vi "2P_AdapUprite_Linlin.vi"() -> ()   [LabVIEW 2015] (continued)
                            n110 = local read "AI channels"() -> (w2310:i32[])
                            n111 = local read "CI channels"() -> (w2309:i32[])
                            n112 = call "2pparameters.vi"("command"="get") -> ("params out"=w2307:T12)  [unwired: 1 in]
                            n113 = Bundle By Name(cluster=w2307, "aAI"=w2310, "aCI"=w2309, "aAS"=w2304) -> (w2308:T12)
                            n114 = call "2pparameters.vi"("Params in"=w2308, "command"="set") -> ()  [unwired: 1 out]
                          }
                          frame #1 {
                            n115 = local read "Vy-min ref"() -> (w2315:dbl)
                            n116 = local read "Vy-max ref"() -> (w2316:dbl)
                            n117 = local read "Angle ref"() -> (w2314:dbl)
                            n118 = local read "Vx-min ref"() -> (w2317:dbl)
                            n119 = local write "counts"(0 ("counts")) -> ()
                            n120 = local write "graphtab"(T8."image" ("graphtab")) -> ()
                            n121 = local read "Vx-max ref"() -> (w2318:dbl)
                            n122 = property on="Stop" class="Bool (strict)"("Visible"=TRUE, "DisabledEnum"=T7."Enabled" ("Disabled")) -> ()  [unwired: 2 in, 2 out]
                            n123 = property on="Start" class="Bool (strict)"("Visible"=FALSE, "DisabledEnum"=T7."Disabled and Grayed Out" ("Disabled")) -> ()  [unwired: 2 in, 2 out]
                            n124 = script code="Xic=(ximax+ximin)./2;\nYic=(yimax+yimin)./2;\nximin=ximin-Xic;\nymin=ymin-Yic;\nxirmin=ximin.*cos(pi/180.*phi)+yimin.*sin(pi./180.*phi)+Xic;\nyirmin=-ximin.*sin(pi./180.*phi)+yimin.*cos(pi./180.*phi)+Yic;"("ximax"=w2318, "ximin"=w2317, "yimax"=w2316, "yimin"=w2315, "phi"=w2314) -> ("xirmin"=w2313:dbl, "yirmin"=w2312:dbl)  [unwired: 1 in, 1 out]
                            n125 = stacked-sequence {
                              tunnel: w2311 -> [_ w2343 _]
                              frame #0 {
                                n126 = local read "Measurement"() -> (w2325:T4)
                                n127 = case shown="\"X-Y-Z stack\"" w2325 {
                                frame "X-Y-t movie", Default {
                                n128 = call "2pparameters.vi"("command"="get") -> ("params out"=w2328:T12)  [unwired: 1 in]
                                n129 = Bundle By Name(cluster=w2328, "type"="X-Y-t movie") -> (w2326:T12)
                                n130 = call "2pparameters.vi"("Params in"=w2326, "command"="set") -> ()  [unwired: 1 out]
                                }
                                frame "X-Y-Z stack" {
                                n131 = call "2pparameters.vi"("command"="get") -> ("params out"=w2333:T12)  [unwired: 1 in]
                                n132 = Bundle By Name(cluster=w2333, "type"="X-Y-Z stack") -> (w2331:T12)
                                n133 = call "2pparameters.vi"("Params in"=w2331, "command"="set") -> ()  [unwired: 1 out]
                                }
                                frame "Lifetime (scan)" {
                                n134 = call "2pparameters.vi"("command"="get") -> ("params out"=w2338:T12)  [unwired: 1 in]
                                n135 = Bundle By Name(cluster=w2338, "type"="Lifetime (scan)") -> (w2336:T12)
                                n136 = call "2pparameters.vi"("Params in"=w2336, "command"="set") -> ()  [unwired: 1 out]
                                }
                                }
                              }
                              frame #1 {
                                n137 = Format Date/Time String(time format string (%c)="%Y%m%d", seconds (now)=w2343) -> (date/time string=w2342:string)  [unwired: 1 in]
                                n138 = Format Date/Time String(time format string (%c)="%H%M%S", seconds (now)=w2343) -> (date/time string=w2341:string)  [unwired: 1 in]
                                n139 = call "2pparameters.vi"("command"="get") -> ("params out"=w2347:T12)  [unwired: 1 in]
                                n140 = Bundle By Name(cluster=w2347, "date"=w2342, "time"=w2341) -> (w2346:T12)
                                n141 = call "2pparameters.vi"("Params in"=w2346, "command"="set") -> ()  [unwired: 1 out]
                              }
                              frame #2 {
                                n142 = call "configuration_2P_Linlin.vi"("command"="get") -> ("config out"=w2350:T14)  [unwired: 2 in, 1 out]
                                n143 = Unbundle By Name(w2350) -> ("CI names"=w2358:string[], "AI names"=w2359:string[])
                                n144 = call "2pparameters.vi"("command"="get") -> ("params out"=w2355:T12)  [unwired: 1 in]
                                n145 = Unbundle By Name(w2355) -> ("aCI"=w2356:i32[], "aAI"=w2357:i32[])
                                n146 = for {
                                tunnel: w2356 -> [w2369] mode=indexing
                                tunnel: w2358 -> [w2370]
                                tunnel: [w2368] -> w2360 mode=indexing
                                n147 = Index Array(array=w2370, index=w2369) -> (element=w2368:string)
                                }
                                n148 = for {
                                tunnel: w2357 -> [w2366] mode=indexing
                                tunnel: w2359 -> [w2367]
                                tunnel: [w2365] -> w2361 mode=indexing
                                n149 = Index Array(array=w2367, index=w2366) -> (element=w2365:string)
                                }
                                n150 = Build Array (concatenate)(w2360, w2361) -> (w2353:string[])
                                n151 = for {
                                tunnel: w2353 -> [w2363] mode=indexing
                                tunnel: [w2362] -> w2352 mode=indexing
                                i -> [w2364]
                                n152 = Bundle("String"=w2363, w2364) -> (w2362:cluster{"String":string, i32})  [unwired: 1 in]
                                }
                                n153 = property on="image2list" class="Ring (strict)"("StringsAndValues[]"=w2352) -> ()  [unwired: 2 in, 2 out]
                                n154 = property on="image1list" class="Ring (strict)"("StringsAndValues[]"=w2352) -> ()  [unwired: 2 in, 2 out]
                                n155 = property on="image1list chB" class="Ring (strict)"("StringsAndValues[]"=w2352) -> ()  [unwired: 2 in, 2 out]
                                n156 = property on="image1list chA" class="Ring (strict)"("StringsAndValues[]"=w2352) -> ()  [unwired: 2 in, 2 out]
                              }
                            }
                            n157 = call "setposition.vi"("Vy"=w2312, "Vx"=w2313) -> ()  [unwired: 1 in]
                          }
                          frame #2 {
                            n158 = call "X-array-databuffer.vi"("command"=enum16{"get", "set", "clear", "append"}."clear") -> ()  [unwired: 3 in, 2 out]
                            n159 = call "Y-array-databuffer.vi"("command"=enum16{"get", "set", "clear", "append"}."clear") -> ()  [unwired: 3 in, 2 out]
                            n160 = call "2pparameters.vi"("command"="get") -> ("params out"=w2374:T12)  [unwired: 1 in]
                            n161 = Unbundle By Name(w2374) -> ("aAS"=w2371:u32[], "autoshutter"=w2375:bool, "auto OD"=w2372:bool)
                            n162 = call "allAI-temp_img.vi"("command"=enum16{"get", "set", "clear", "append"}."clear") -> ()  [unwired: 3 in, 2 out]
                            n163 = case shown="True" w2372 {
                              frame False {
                              }
                              frame True {
                                n164 = call "configuration_2P_Linlin.vi"("command"="get") -> ("config out"=w2381:T14)  [unwired: 2 in, 1 out]
                                n165 = Unbundle By Name(w2381) -> ("image OD"=w2384:u16)
                                n166 = local read "ODfilt"() -> (w2383:u16)
                                n167 = call "filterwheelcontrol_nothorlabslib.vi"("Current OD filt"=w2383, "New ODfilt"=w2384) -> ()  [unwired: 1 in]
                              }
                            }
                            n168 = case shown="True" w2375 {
                              tunnel: w2371 -> [_ w2385]
                              frame False {
                              }
                              frame True {
                                n169 = call "shuttercontrol_multi.vi"("Autoshutter Chans"=w2385, "command"="close") -> ()  [unwired: 1 in, 1 out]
                              }
                            }
                            n170 = call "CH1-temp.vi"("command"=enum16{"get", "set", "clear", "add row"}."clear") -> ()  [unwired: 3 in, 2 out]
                            n171 = call "CH2-temp.vi"("command"=enum16{"get", "set", "clear", "add row"}."clear") -> ()  [unwired: 3 in, 2 out]
                          }
                          frame #3 {
                            n172 = local read "avpp"() -> (w2419:i32)
                            n173 = local read "Angle ref"() -> (w2418:dbl)
                            n174 = local read "ROI Type"() -> (w2417:u16)
                            n175 = local read "xpixels ref"() -> (w2414:i32)
                            n176 = local read "Vx-min ref"() -> (w2413:dbl)
                            n177 = local read "Vx-max ref"() -> (w2412:dbl)
                            n178 = local read "ypixels ref"() -> (w2410:i32)
                            n179 = local read "Vy-min ref"() -> (w2411:dbl)
                            n180 = local read "Vy-max ref"() -> (w2407:dbl)
                            n181 = local read "Sampling rate"() -> (w2401:dbl)
                            n182 = local read "finite samples"() -> (w2402:bool)
                            n183 = local read "continuous"() -> (w2405:bool)
                            n184 = local read "wavdet"() -> (w2406:bool)
                            n185 = local read "# of frames"() -> (w2404:i32)
                            n186 = local read "maxbufferAI"() -> (w2403:i32)
                            n187 = local read "Override AI buffer"() -> (w2387:bool)
                            n188 = call "2pparameters.vi"("command"="get") -> ("params out"=w2416:T12)  [unwired: 1 in]
                            n189 = Bundle By Name(cluster=w2416, "avpp"=w2419, "Angle Img"=w2418, "Xpixels Img"=w2414, "Vx-min Img"=w2413, "VX-max Img"=w2412, "Ypixels Img"=w2410, "Vy-min Img"=w2411, "Vy-max Img"=w2407, "srate"=w2401, "srate Img"=w2401, "finite"=w2402, "cont"=w2405, "wavdet"=w2406, "measpoints"=w2404, "maxbufferAI"=w2403, "Drawing Mode"=w2417, "Vz-reset"=0.0, "AIoverride"=w2387) -> (w2408:T12)
                            n190 = call "2pparameters.vi"("Params in"=w2408, "command"="set") -> ()  [unwired: 1 out]
                            n191 = local read "Vholding (mV)"() -> (w2390:sgl)
                            n192 = local read "OCgain"() -> (w2391:sgl)
                            n193 = local read "holdon"() -> (w2389:bool)
                            n194 = local read "Current Clamp"() -> (w2396:bool)
                            n195 = local read "Voltage Clamp"() -> (w2395:bool)
                            n196 = local read "CC_ICgain"() -> (w2394:dbl)
                            n197 = call "patchparameters.vi"("command"="get") -> ("Params out"=w2398:T16)  [unwired: 1 in]
                            n198 = Bundle By Name(cluster=w2398, "VC"=w2395, "CC"=w2396, "CC_icg (pA/mv)"=w2394, "VC_icg (mV/mV)"=sgl 10.0, "OCG (mV/pA)"=w2391, "OVG (mV/mV)"=0.1, "Vhold (mV)"=w2390, "holdon"=w2389) -> (w2397:T16)
                            n199 = call "patchparameters.vi"("Params in"=w2397, "command"="set") -> ()  [unwired: 1 out]
                          }
                          frame #4 {
                            # "these store the actual scanning waveforms (for one iteration)"
                            # "Generate Waveforms for Scanning Mirrors"
                            # "Creates The scanning waveform here"
                            n200 = call "2pparameters.vi"("command"="get") -> ("params out"=w2434:T12)  [unwired: 1 in]
                            n201 = Unbundle By Name(w2434) -> ("srate Img"=w2433:sgl, "Angle Img"=w2432:dbl, "VX-max Img"=w2431:dbl, "Vx-min Img"=w2430:dbl, "Xpixels Img"=w2429:i32, "Ypixels Img"=w2428:i32, "Vy-max Img"=w2427:dbl, "Vy-min Img"=w2426:dbl, "Drawing Mode"=w2425:u16)
                            n202 = call "ROI-databuffer.vi"("command"=enum16{"get", "set", "clear", "append"}."get") -> ("array out"=w2424:cluster{"x":sgl, "y":sgl}[])  [unwired: 4 in]
                            n203 = call "ScanningWaveform_v4.vi"("Vy-min"=w2426, "Vy-max"=w2427, "yPixels/tPixels"=w2428, "xPixels/rPixels"=w2429, "Vx-min"=w2430, "Vx-max"=w2431, "Drawing Mode"=w2425, "Angle"=w2432, "AOrate"=w2433, "Points"=w2424) -> ("numPixels"=w2420:dbl, "Y-WaveArray"=w2423:dbl[], "P"=w2421:dbl, "X-WaveArray"=w2422:dbl[])  [unwired: 6 in]
                            n204 = call "2pparameters.vi"("command"="get") -> ("params out"=w2442:T12)  [unwired: 1 in]
                            n205 = call "Y-array-databuffer.vi"("array in"=w2423, "command"=enum16{"get", "set", "clear", "append"}."set") -> ()  [unwired: 2 in, 2 out]
                            n206 = call "X-array-databuffer.vi"("array in"=w2422, "command"=enum16{"get", "set", "clear", "append"}."set") -> ()  [unwired: 2 in, 2 out]
                            n207 = Bundle By Name(cluster=w2442, "P"=w2421, "sAOxy"=w2420) -> (w2439:T12)
                            n208 = call "2pparameters.vi"("Params in"=w2439, "command"="set") -> ()  [unwired: 1 out]
                          }
                          frame #5 {
                            # "rem2Ps"
                            # "A2Ps"
                            # "Al"
                            # "Rl"
                            # "Combines scanning waveform with \"wavform generation\" waveforms"
                            n209 = stacked-sequence {
                              seq-local: [w2461 _ _ _ _ _ _ _ _ _ _] -> [_ w2581 _ w2636 _ w2716 _ _ _ _ _]
                              seq-local: [w2462 _ _ _ _ _ _ _ _ _ _] -> [_ w2582 w2592 _ w2685 _ _ _ _ _ _]
                              seq-local: [_ _ w2591 _ _ _ _ _ _ _ _] -> [_ _ _ _ w2679 _ _ _ _ _ _]
                              seq-local: [_ _ _ w2635 _ _ _ _ _ _ _] -> [_ _ _ _ _ w2715 _ _ _ _ _]
                              seq-local: [w2458 _ _ _ _ _ _ _ _ _ _] -> [_ w2578 _ _ _ _ _ _ w2925 w2993 _]
                              seq-local: [w2457 _ _ _ _ _ _ _ _ _ _] -> [_ w2577 _ _ _ _ _ _ w2926 w2994 _]
                              seq-local: [w2464 _ _ _ _ _ _ _ _ _ _] -> [_ _ _ _ _ _ w2754 _ w2924 w2992 _]
                              seq-local: [w2460 _ _ _ _ _ _ _ _ _ _] -> [_ w2576 _ _ _ _ w2753 w2832 _ _ _]
                              seq-local: [w2459 _ _ _ _ _ _ _ _ _ _] -> [_ w2575 _ _ _ _ w2752 w2831 _ _ _]
                              seq-local: [w2463 _ _ _ _ _ _ _ _ _ _] -> [_ _ _ _ _ _ w2751 w2830 _ _ _]
                              tunnel: [_ _ w2590 _ _ _ _ _ _ _ _] -> w2455
                              tunnel: [_ _ w2589 _ _ _ _ _ _ _ _] -> w2454
                              tunnel: [w2462 _ _ _ _ _ _ _ _ _ _] -> w2456
                              tunnel: [w2461 _ _ _ _ _ _ _ _ _ _] -> w2453
                              tunnel: [_ _ _ w2634 _ _ _ _ _ _ _] -> w2452
                              tunnel: [_ _ _ w2633 _ _ _ _ _ _ _] -> w2451
                              tunnel: [w2460 _ _ _ _ _ _ _ _ _ _] -> w2450
                              tunnel: [w2459 _ _ _ _ _ _ _ _ _ _] -> w2449
                              tunnel: [_ _ _ _ _ _ w2750 _ _ _ _] -> w2448
                              tunnel: [_ _ _ _ _ _ _ w2829 _ _ _] -> w2447
                              tunnel: [w2458 _ _ _ _ _ _ _ _ _ _] -> w2446
                              tunnel: [w2457 _ _ _ _ _ _ _ _ _ _] -> w2445
                              tunnel: [_ _ _ _ _ _ _ _ w2923 _ _] -> w2444
                              tunnel: [_ _ _ _ _ _ _ _ _ w2991 _] -> w2443
                              frame #0 {
                                # "channels\nadded/removed"
                                # "all these arrows go to frames\n6 and 7"
                                # "for a next version, give ome thought to\nthe possibilit of intermittently updating the\nwaveforms. it will have to be a calculation\nbased on speed of CPU and program on the one hand\nand length of measurement on the other. but then it should be possible, in principle, to \nupdate the waveform on the fly and that way cut up a longer measurement in smaller parts."
                                # "Y"
                                # "X"
                                # "This frame takes channels from \"waveform generation\" and adds, X,Y,2p shutter and Lifetime Timestamp (if those where not manually defined in WG)"
                                n210 = stacked-sequence {
                                tunnel: [w2467 _ _ _] -> w2462
                                tunnel: [_ w2479 _ _] -> w2461
                                tunnel: [_ _ _ w2542] -> w2457
                                tunnel: [_ _ _ w2541] -> w2458
                                tunnel: [_ _ _ w2540] -> w2464
                                tunnel: [_ _ w2492 _] -> w2460
                                tunnel: [_ _ w2491 _] -> w2459
                                tunnel: [_ _ w2490 _] -> w2463
                                frame #0 {
                                n211 = call "configuration_2P_Linlin.vi"("command"="get") -> ("config out"=w2465:T14)  [unwired: 2 in, 1 out]
                                n212 = Unbundle By Name(w2465) -> ("Voltage to Xgalvo"=w2468:i32)
                                n213 = call "2pparameters.vi"("command"="get") -> ("params out"=w2471:T12)  [unwired: 1 in]
                                n214 = in-place {
                                in-place-border: w2468 -> [w2476]
                                in-place-border: [w2473] -> w2467
                                n215 = in-place-cluster #1(w2471) -> ("aAO"=w2475:u32[])
                                n216 = call "add channel to active arrayv2.vi"("line array in"=w2475, "line to add"=w2476) -> ("line array out"=w2474:u32[], "addition"=w2473:bool)  [unwired: 1 out]
                                n217 = in-place-cluster #1("aAO"=w2474) -> (w2469:T12)
                                }
                                n218 = call "2pparameters.vi"("Params in"=w2469, "command"="set") -> ()  [unwired: 1 out]
                                }
                                frame #1 {
                                n219 = call "configuration_2P_Linlin.vi"("command"="get") -> ("config out"=w2477:T14)  [unwired: 2 in, 1 out]
                                n220 = Unbundle By Name(w2477) -> ("Voltage to Ygalvo"=w2480:i32)
                                n221 = call "2pparameters.vi"("command"="get") -> ("params out"=w2483:T12)  [unwired: 1 in]
                                n222 = in-place {
                                in-place-border: w2480 -> [w2488]
                                in-place-border: [w2485] -> w2479
                                n223 = in-place-cluster #2(w2483) -> ("aAO"=w2487:u32[])
                                n224 = call "add channel to active arrayv2.vi"("line array in"=w2487, "line to add"=w2488) -> ("line array out"=w2486:u32[], "addition"=w2485:bool)  [unwired: 1 out]
                                n225 = in-place-cluster #2("aAO"=w2486) -> (w2481:T12)
                                }
                                n226 = call "2pparameters.vi"("Params in"=w2481, "command"="set") -> ()  [unwired: 1 out]
                                }
                                frame #2 {
                                n227 = call "2pparameters.vi"("command"="get") -> ("params out"=w2494:T12)  [unwired: 1 in]
                                n228 = Unbundle By Name(w2494) -> ("autoshutter"=w2493:bool, "wavdet"=w2489:bool)
                                n229 = case shown="False" w2493 {
                                tunnel: [w2499 w2522] -> w2492
                                tunnel: [w2498 FALSE ("removal")] -> w2491
                                tunnel: [w2497 w2521] -> w2490
                                tunnel: w2489 -> [w2496 _]
                                frame False {
                                n230 = case shown="False" w2496 {
                                tunnel: [FALSE ("addition") FALSE ("addition")] -> w2499
                                tunnel: [w2503 FALSE ("removal")] -> w2498
                                tunnel: [w2502 _] -> w2497
                                frame False {
                                n231 = call "2pparameters.vi"("command"="get") -> ("params out"=w2501:T12)  [unwired: 1 in]
                                n232 = Unbundle By Name(w2501) -> ("aAS"=w2500:u32[])
                                n233 = in-place {
                                in-place-border: [w2508] -> w2503
                                in-place-border: [w2511] -> w2502
                                in-place-border: w2500 -> [w2510]
                                n234 = in-place-cluster #3(w2501) -> ("aDO"=w2513:u32[])
                                n235 = for {
                                tunnel: [w2516] -> w2509 mode=indexing
                                tunnel: [w2515] -> w2511 mode=indexing
                                shift-right: [w2517] -> w2512
                                shift-left: w2513 -> [w2518]
                                tunnel: w2510 -> [w2514] mode=indexing
                                n236 = call "remove channel from active arrayv2.vi"("line array in"=w2518, "line to remove"=w2514) -> ("line array out"=w2517:u32[], "removal"=w2516:bool, "index"=w2515:i32)
                                }
                                n237 = Or Array Elements(Boolean array=w2509) -> (logical OR=w2508:bool)
                                n238 = in-place-cluster #3("aDO"=w2512) -> (w2504:T12)
                                }
                                n239 = call "2pparameters.vi"("Params in"=w2504, "command"="set") -> ()  [unwired: 1 out]
                                }
                                frame True {
                                }
                                }
                                }
                                frame True {
                                n240 = call "2pparameters.vi"("command"="get") -> ("params out"=w2524:T12)  [unwired: 1 in]
                                n241 = Unbundle By Name(w2524) -> ("aAS"=w2523:u32[])
                                n242 = in-place {
                                in-place-border: w2523 -> [w2534]
                                in-place-border: [w2530] -> w2522
                                in-place-border: [w2529] -> w2521
                                n243 = in-place-cluster #4(w2524) -> ("aDO"=w2533:u32[])
                                n244 = for {
                                tunnel: w2534 -> [w2539] mode=indexing
                                shift-right: [w2537] -> w2532
                                shift-left: w2533 -> [w2538]
                                tunnel: [w2536] -> w2531 mode=indexing
                                tunnel: [w2535] -> w2529 mode=indexing
                                n245 = call "add channel to active arrayv2.vi"("line array in"=w2538, "line to add"=w2539) -> ("line array out"=w2537:u32[], "addition"=w2536:bool, "index"=w2535:i32)
                                }
                                n246 = Or Array Elements(Boolean array=w2531) -> (logical OR=w2530:bool)
                                n247 = in-place-cluster #4("aDO"=w2532) -> (w2526:T12)
                                }
                                n248 = call "2pparameters.vi"("Params in"=w2526, "command"="set") -> ()  [unwired: 1 out]
                                }
                                }
                                }
                                frame #3 {
                                n249 = local read "Measurement"() -> (w2543:T4)
                                n250 = To Unsigned Long Integer(number=w2543) -> (unsigned 32bit integer=w2544:u32)
                                n251 = case shown="5..7" w2544 {
                                tunnel: [FALSE ("addition") w2564] -> w2542
                                tunnel: [w2549 FALSE ("removal")] -> w2541
                                tunnel: [w2547 w2562] -> w2540
                                frame 0..4, Default {
                                n252 = call "configuration_2P_Linlin.vi"("command"="get") -> ("config out"=w2545:T14)  [unwired: 2 in, 1 out]
                                n253 = Unbundle By Name(w2545) -> ("LT timestamp"=w2552:u32)
                                n254 = call "2pparameters.vi"("command"="get") -> ("params out"=w2553:T12)  [unwired: 1 in]
                                n255 = in-place {
                                in-place-border: w2552 -> [w2559]
                                in-place-border: [w2556] -> w2549
                                in-place-border: [w2555] -> w2547
                                n256 = in-place-cluster #5(w2553) -> ("aDO"=w2558:u32[])
                                n257 = call "remove channel from active arrayv2.vi"("line array in"=w2558, "line to remove"=w2559) -> ("line array out"=w2557:u32[], "removal"=w2556:bool, "index"=w2555:i32)
                                n258 = in-place-cluster #5("aDO"=w2557) -> (w2550:T12)
                                }
                                n259 = call "2pparameters.vi"("Params in"=w2550, "command"="set") -> ()  [unwired: 1 out]
                                }
                                frame 5..7 {
                                n260 = call "configuration_2P_Linlin.vi"("command"="get") -> ("config out"=w2560:T14)  [unwired: 2 in, 1 out]
                                n261 = Unbundle By Name(w2560) -> ("LT timestamp"=w2567:u32)
                                n262 = call "2pparameters.vi"("command"="get") -> ("params out"=w2568:T12)  [unwired: 1 in]
                                n263 = in-place {
                                in-place-border: w2567 -> [w2574]
                                in-place-border: [w2571] -> w2564
                                in-place-border: [w2570] -> w2562
                                n264 = in-place-cluster #6(w2568) -> ("aDO"=w2573:u32[])
                                n265 = call "add channel to active arrayv2.vi"("line array in"=w2573, "line to add"=w2574) -> ("line array out"=w2572:u32[], "addition"=w2571:bool, "index"=w2570:i32)
                                n266 = in-place-cluster #6("aDO"=w2572) -> (w2565:T12)
                                }
                                n267 = call "2pparameters.vi"("Params in"=w2565, "command"="set") -> ()  [unwired: 1 out]
                                }
                                }
                                }
                                }
                              }
                              frame #1 {
                                # "Prepares the actual AO and DO lines that are going to be used for the task"
                                n268 = Or(x=w2581, y=w2582) -> (x .or. y?=w2580:bool)
                                n269 = case shown="True" w2580 {
                                frame False {
                                }
                                frame True {
                                # "update GUI"
                                n270 = call "Used AO lines.vi"() -> ("used AO names"=w2586:string[], "used AO lines"=w2588:tag[])  [unwired: 2 in]
                                n271 = control-ref of="Analog Lines Plot"() -> (w2587:refnum<vi>)
                                n272 = local write "Analog Used Lines"(w2588) -> ()
                                n273 = local write "Analog Used Names"(w2586) -> ()
                                n274 = call "prepAOWaveplot.vi"("WaveformGraph in"=w2587, "Analog Used Names"=w2586) -> ()  [unwired: 1 in]
                                }
                                }
                                n275 = Compound Arithmetic op=OR(w2578, w2577, w2576, w2575) -> (w2579:bool)
                                n276 = case shown="True" w2579 {
                                frame False {
                                }
                                frame True {
                                n277 = control-ref of="Digital Lines Plot"() -> (w2583:refnum<vi>)
                                n278 = call "Used DO lines.vi"() -> ("used DO names"=w2584:string[], "used DO lines"=w2585:tag[])  [unwired: 2 in]
                                n279 = local write "Digital Used Lines"(w2585) -> ()
                                n280 = local write "Digital Used Names"(w2584) -> ()
                                n281 = call "prepDOWaveplot.vi"("DigitalGraph in"=w2583, "used DO names"=w2584) -> ()  [unwired: 1 in]
                                }
                                }
                              }
                              frame #2 {
                                # "Make sure that the parameters used to create waveform are saved in the right format"
                                n282 = case shown="True" w2592 {
                                tunnel: [w2595 w2618] -> w2591
                                tunnel: [w2594 w2616] -> w2590
                                tunnel: [w2593 _] -> w2589
                                frame False {
                                n283 = stacked-sequence {
                                seq-local: [w2599 _] -> [_ w2610]
                                tunnel: [w2599 _] -> w2595
                                tunnel: [w2602 _] -> w2594
                                tunnel: [w2598 _] -> w2593
                                frame #0 {
                                n284 = call "configuration_2P_Linlin.vi"("command"="get") -> ("config out"=w2596:T14)  [unwired: 2 in, 1 out]
                                n285 = call "waveformparamsv2.vi"("command"="get") -> ("Params out"=w2604:T17)  [unwired: 4 in, 2 out]
                                n286 = Unbundle By Name(w2596) -> ("Voltage to Xgalvo"=w2609:i32)
                                n287 = call "2pparameters.vi"("command"="get") -> ("params out"=w2607:T12)  [unwired: 1 in]
                                n288 = Unbundle By Name(w2604) -> ("AO parameters"=w2603:T18)
                                n289 = Unbundle By Name(w2607) -> ("aAO"=w2608:u32[])
                                n290 = call "waveformsAObuffer.vi"("command"="get") -> ("AO wf out"=w2600:waveform(dbl)[])  [unwired: 1 in]
                                n291 = Search 1D Array(1D array=w2608, element=w2609) -> (index of element=w2599:i32)  [unwired: 1 in]
                                n292 = Index Array(array=w2600, index=w2599) -> (element=w2598:waveform(dbl))
                                n293 = Index Array(array=w2603, index=w2599) -> (element=w2602:T19)
                                }
                                frame #1 {
                                w2611 = 0.0 ("Step size (V)")
                                n294 = local read "Sampling rate"() -> (w2612:dbl)
                                n295 = call "replace AO XYwfparam.vi"("Baseline (V)"=w2611, "Start amplitude (V)"=w2611, "Cycles"=w2611, "Repeats"=w2611, "index of AO wave"=w2610, "Step size (V)"=w2611, "DC (%)"=w2611, "Sampling frequency (Hz)"=w2612, "Period (ms)"=w2611, "Cycle length (s)"=w2611, "Pulses"=w2611, "padding value"=w2611, "Matlab wave name"=path "xwave") -> ()  [unwired: 3 in]
                                }
                                }
                                }
                                frame True {
                                w2617 = 0.0 ("Repeats")
                                n296 = local read "Sampling rate"() -> (w2624:dbl)
                                n297 = call "2pparameters.vi"("command"="get") -> ("params out"=w2620:T12)  [unwired: 1 in]
                                n298 = call "waveformparamsv2.vi"("command"="get") -> ("Params out"=w2630:T17)  [unwired: 4 in, 2 out]
                                n299 = call "configuration_2P_Linlin.vi"("command"="get") -> ("config out"=w2614:T14)  [unwired: 2 in, 1 out]
                                n300 = Unbundle By Name(w2614) -> ("Voltage to Xgalvo"=w2622:i32)
                                n301 = Unbundle By Name(w2630) -> ("AO parameters"=w2627:T18)
                                n302 = Unbundle By Name(w2620) -> ("aAO"=w2621:u32[])
                                n303 = Search 1D Array(1D array=w2621, element=w2622) -> (index of element=w2618:i32)  [unwired: 1 in]
                                n304 = Index Array(array=w2627, index=0) -> (element=w2628:T19)
                                n305 = Bundle By Name(cluster=w2628, "AOtab"=-1.0 ("Repeats"), "Repeats"=w2617, "Cycles"=w2617, "Start amplitude (V)"=w2617, "Baseline (V)"=w2617, "Step size (V)"=w2617, "DC (%)"=w2617, "Sampling frequency (Hz)"=w2624, "Period (ms)"=w2617, "Offset (V)"=w2617, "Amplitude (V)"=w2617, "Frequency"=w2617, "Tri Repeats"=w2617, "phase shift (ms)"=w2617, "Pulses"=w2617, "Matlab wave file"=path "xwave", "padding value"=w2617) -> (w2616:T19)
                                n306 = Build Array(w2616) -> (w2625:T18)
                                n307 = call "waveformparamsv2.vi"("command"="add AO", "add AO"=w2625) -> ()  [unwired: 3 in, 3 out]
                                }
                                }
                              }
                              frame #3 {
                                n308 = case shown="True" w2636 {
                                tunnel: [w2639 w2662] -> w2635
                                tunnel: [w2638 w2660] -> w2634
                                tunnel: [w2637 _] -> w2633
                                frame False {
                                n309 = stacked-sequence {
                                seq-local: [w2643 _] -> [_ w2654]
                                tunnel: [w2643 _] -> w2639
                                tunnel: [w2646 _] -> w2638
                                tunnel: [w2642 _] -> w2637
                                frame #0 {
                                n310 = call "configuration_2P_Linlin.vi"("command"="get") -> ("config out"=w2640:T14)  [unwired: 2 in, 1 out]
                                n311 = call "waveformparamsv2.vi"("command"="get") -> ("Params out"=w2648:T17)  [unwired: 4 in, 2 out]
                                n312 = Unbundle By Name(w2640) -> ("Voltage to Ygalvo"=w2653:i32)
                                n313 = call "2pparameters.vi"("command"="get") -> ("params out"=w2651:T12)  [unwired: 1 in]
                                n314 = Unbundle By Name(w2648) -> ("AO parameters"=w2647:T18)
                                n315 = Unbundle By Name(w2651) -> ("aAO"=w2652:u32[])
                                n316 = call "waveformsAObuffer.vi"("command"="get") -> ("AO wf out"=w2644:waveform(dbl)[])  [unwired: 1 in]
                                n317 = Search 1D Array(1D array=w2652, element=w2653) -> (index of element=w2643:i32)  [unwired: 1 in]
                                n318 = Index Array(array=w2644, index=w2643) -> (element=w2642:waveform(dbl))
                                n319 = Index Array(array=w2647, index=w2643) -> (element=w2646:T19)
                                }
                                frame #1 {
                                w2655 = 0.0 ("Step size (V)")
                                n320 = local read "Sampling rate"() -> (w2656:dbl)
                                n321 = call "replace AO XYwfparam.vi"("Baseline (V)"=w2655, "Start amplitude (V)"=w2655, "Cycles"=w2655, "Repeats"=w2655, "index of AO wave"=w2654, "Step size (V)"=w2655, "DC (%)"=w2655, "Sampling frequency (Hz)"=w2656, "Period (ms)"=w2655, "Cycle length (s)"=w2655, "Pulses"=w2655, "padding value"=w2655, "Matlab wave name"=path "ywave") -> ()  [unwired: 3 in]
                                }
                                }
                                }
                                frame True {
                                w2661 = 0.0 ("Repeats")
                                n322 = local read "Sampling rate"() -> (w2669:dbl)
                                n323 = call "configuration_2P_Linlin.vi"("command"="get") -> ("config out"=w2658:T14)  [unwired: 2 in, 1 out]
                                n324 = call "2pparameters.vi"("command"="get") -> ("params out"=w2664:T12)  [unwired: 1 in]
                                n325 = call "waveformparamsv2.vi"("command"="get") -> ("Params out"=w2675:T17)  [unwired: 4 in, 2 out]
                                n326 = Unbundle By Name(w2658) -> ("Voltage to Ygalvo"=w2666:i32)
                                n327 = Unbundle By Name(w2675) -> ("AO parameters"=w2672:T18)
                                n328 = Unbundle By Name(w2664) -> ("aAO"=w2665:u32[])
                                n329 = Search 1D Array(1D array=w2665, element=w2666) -> (index of element=w2662:i32)  [unwired: 1 in]
                                n330 = Index Array(array=w2672, index=0) -> (element=w2673:T19)
                                n331 = Bundle By Name(cluster=w2673, "AOtab"=-1.0 ("Repeats"), "Repeats"=w2661, "Cycles"=w2661, "Start amplitude (V)"=w2661, "Baseline (V)"=w2661, "Step size (V)"=w2661, "DC (%)"=w2661, "Sampling frequency (Hz)"=w2669, "Period (ms)"=w2661, "Offset (V)"=w2661, "Amplitude (V)"=w2661, "Frequency"=w2661, "Tri Repeats"=w2661, "phase shift (ms)"=w2661, "Pulses"=w2661, "Matlab wave file"=path "ywave", "padding value"=w2661) -> (w2660:T19)
                                n332 = Build Array(w2660) -> (w2670:T18)
                                n333 = call "waveformparamsv2.vi"("command"="add AO", "add AO"=w2670) -> ()  [unwired: 3 in, 3 out]
                                }
                                }
                              }
                              frame #4 {
                                # "Create waveforms for X"
                                n334 = call "2pparameters.vi"("command"="get") -> ("params out"=w2682:T12)  [unwired: 1 in]
                                n335 = Unbundle By Name(w2682) -> ("wavdet"=w2681:bool, "sAOxy"=w2678:i32, "refwfsize"=w2677:dbl, "srate Img"=w2680:sgl)
                                n336 = case shown="True" w2681 {
                                tunnel: [w2686 w2696] -> w2684
                                tunnel: w2680 -> [w2687 w2698]
                                tunnel: w2678 -> [_ w2694]
                                tunnel: w2677 -> [_ w2693]
                                frame False {
                                n337 = call "X-array-databuffer.vi"("command"=enum16{"get", "set", "clear", "append"}."get") -> ("array out"=w2690:dbl[])  [unwired: 3 in, 1 out]
                                n338 = Reciprocal(x=w2687) -> (1/x=w2688:sgl)
                                n339 = Bundle By Name("Y"=w2690, "dt"=w2688) -> (w2686:waveform(dbl))  [unwired: 1 in]
                                }
                                frame True {
                                n340 = To Double Precision Float(number=w2694) -> (double precision float=w2695:dbl)
                                n341 = Divide(x=w2693, y=w2695) -> (x/y=w2691:dbl)
                                n342 = Round Toward +Infinity(x=w2691) -> (ceil(x): smallest int >= x=w2692:dbl)
                                n343 = call "X-array-databuffer.vi"("command"=enum16{"get", "set", "clear", "append"}."get") -> ("array out"=w2700:dbl[])  [unwired: 3 in, 1 out]
                                n344 = Reciprocal(x=w2698) -> (1/x=w2699:sgl)
                                n345 = for {
                                N: w2692 -> [_]
                                tunnel: w2700 -> [w2702]
                                tunnel: [w2702] -> w2697 mode=concatenating
                                }
                                n346 = Bundle By Name("Y"=w2697, "dt"=w2699) -> (w2696:waveform(dbl))  [unwired: 1 in]
                                }
                                }
                                n347 = case shown="True" w2685 {
                                tunnel: w2684 -> [w2704 w2710]
                                tunnel: w2679 -> [w2705 _]
                                frame False {
                                n348 = call "waveformsAObuffer.vi"("command"="get") -> ("AO wf out"=w2708:waveform(dbl)[])  [unwired: 1 in]
                                n349 = Replace Array Subset(array=w2708, new element=w2704, index=w2705) -> (w2703:waveform(dbl)[])
                                n350 = call "waveformsAObuffer.vi"("AO wf in"=w2703, "command"="set") -> ()  [unwired: 1 out]
                                }
                                frame True {
                                n351 = call "waveformsAObuffer.vi"("command"="get") -> ("AO wf out"=w2712:waveform(dbl)[])  [unwired: 1 in]
                                n352 = Build Array (concatenate)(w2712, w2710) -> (w2709:waveform(dbl)[])
                                n353 = call "waveformsAObuffer.vi"("AO wf in"=w2709, "command"="set") -> ()  [unwired: 1 out]
                                }
                                }
                              }
                              frame #5 {
                                # "... and create waveform for Y"
                                n354 = call "2pparameters.vi"("command"="get") -> ("params out"=w2724:T12)  [unwired: 1 in]
                                n355 = Unbundle By Name(w2724) -> ("wavdet"=w2723:bool, "sAOxy"=w2721:i32, "refwfsize"=w2722:dbl, "srate Img"=w2717:sgl)
                                n356 = To Double Precision Float(number=w2721) -> (double precision float=w2720:dbl)
                                n357 = Divide(x=w2722, y=w2720) -> (x/y=w2719:dbl)
                                n358 = Round Toward +Infinity(x=w2719) -> (ceil(x): smallest int >= x=w2718:dbl)
                                n359 = case shown="False" w2723 {
                                tunnel: [w2728 w2733] -> w2714
                                tunnel: w2718 -> [_ w2737]
                                tunnel: w2717 -> [w2729 w2735]
                                frame False {
                                n360 = call "Y-array-databuffer.vi"("command"=enum16{"get", "set", "clear", "append"}."get") -> ("array out"=w2726:dbl[])  [unwired: 3 in, 1 out]
                                n361 = Reciprocal(x=w2729) -> (1/x=w2730:sgl)
                                n362 = Bundle By Name("Y"=w2726, "dt"=w2730) -> (w2728:waveform(dbl))  [unwired: 1 in]
                                }
                                frame True {
                                # "Tile the waveform N times if wavefrom generation is being used"
                                n363 = call "Y-array-databuffer.vi"("command"=enum16{"get", "set", "clear", "append"}."get") -> ("array out"=w2731:dbl[])  [unwired: 3 in, 1 out]
                                n364 = Reciprocal(x=w2735) -> (1/x=w2736:sgl)
                                n365 = for {
                                N: w2737 -> [_]
                                tunnel: w2731 -> [w2738]
                                tunnel: [w2738] -> w2734 mode=concatenating
                                }
                                n366 = Bundle By Name("Y"=w2734, "dt"=w2736) -> (w2733:waveform(dbl))  [unwired: 1 in]
                                }
                                }
                                n367 = case shown="False" w2716 {
                                tunnel: w2714 -> [w2741 w2746]
                                tunnel: w2715 -> [w2742 _]
                                frame False {
                                # "Add (tiled) waveform to the full set of waveforms forAO"
                                n368 = call "waveformsAObuffer.vi"("command"="get") -> ("AO wf out"=w2744:waveform(dbl)[])  [unwired: 1 in]
                                n369 = Replace Array Subset(array=w2744, new element=w2741, index=w2742) -> (w2739:waveform(dbl)[])
                                n370 = call "waveformsAObuffer.vi"("AO wf in"=w2739, "command"="set") -> ()  [unwired: 1 out]
                                }
                                frame True {
                                n371 = call "waveformsAObuffer.vi"("command"="get") -> ("AO wf out"=w2748:waveform(dbl)[])  [unwired: 1 in]
                                n372 = Build Array (concatenate)(w2748, w2746) -> (w2745:waveform(dbl)[])
                                n373 = call "waveformsAObuffer.vi"("AO wf in"=w2745, "command"="set") -> ()  [unwired: 1 out]
                                }
                                }
                              }
                              frame #6 {
                                # "Calculate  waveform for the 2p shutter to the digital waveforms (4 possibilities of whether it is there and if it needs to be there)"
                                n374 = Build Array(w2753, w2752) -> (w2756:bool[])
                                n375 = Boolean Array To Number(Boolean array=w2756) -> (number=w2755:u32)
                                n376 = case shown="0" w2755 {
                                tunnel: w2754 -> [_ _ _ _]
                                tunnel: w2751 -> [w2760 w2781 _ w2799]
                                tunnel: [_ w2780 _ w2797] -> w2750
                                frame 1 {
                                w2770 = 0.0 ("DOtab")
                                # "remove True; add False"
                                n377 = call "2pparameters.vi"("command"="get") -> ("params out"=w2767:T12)  [unwired: 1 in]
                                n378 = call "waveformparamsv2.vi"("command"="get") -> ("Params out"=w2776:T17)  [unwired: 4 in, 2 out]
                                n379 = Unbundle By Name(w2776) -> ("DO parameters"=w2774:T20)
                                n380 = Unbundle By Name(w2767) -> ("srate"=w2763:sgl, "sAOxy"=w2766:i32)
                                n381 = To Double Precision Float(number=w2763) -> (double precision float=w2761:dbl)
                                n382 = To Double Precision Float(number=w2763) -> (double precision float=w2762:dbl)
                                n383 = To Double Precision Float(number=w2766) -> (double precision float=w2765:dbl)
                                n384 = Divide(x=w2762, y=w2765) -> (x/y=w2764:dbl)
                                n385 = Index Array(array=w2774, index=0) -> (element=w2773:T21)
                                n386 = Bundle By Name(cluster=w2773, "Digital DC (%)"=100.0, "Digital phase"=w2770, "Digital Freq (Hz)"=w2764, "Sampling frequency (Hz)"=w2761, "Digital time offset (s)"=w2770, "padding value"=0.0, "matlab wave file"=path "2Pshutter", "DOtab"=0.0) -> (w2759:T21)
                                n387 = Array Size(array=w2760) -> (size(s)=w2758:i32)
                                n388 = Initialize Array(w2759, w2758) -> (w2757:T20)
                                n389 = call "waveformparamsv2.vi"("command"="add DO", "add DO"=w2757) -> ()  [unwired: 3 in, 3 out]
                                }
                                frame 2 {
                                # "remove False; add True"
                                n390 = call "waveformparamsv2.vi"("command"="get") -> ("Params out"=w2783:T17)  [unwired: 4 in, 2 out]
                                n391 = in-place {
                                in-place-border: w2781 -> [w2787]
                                in-place-border: [w2786] -> w2780
                                n392 = in-place-cluster #7(w2783) -> ("DO parameters"=w2789:T20)
                                n393 = for {
                                tunnel: w2787 -> [w2793] mode=indexing
                                tunnel: [w2790] -> w2786 mode=indexing
                                shift-right: [w2794] -> w2788
                                shift-left: w2789 -> [w2795]
                                n394 = Delete From Array(array=w2795, length=1, index=w2793) -> (deleted portion=w2792:T20, array with subset deleted=w2794:T20)
                                n395 = Index Array(array=w2792, index=0) -> (element=w2790:T21)
                                }
                                n396 = in-place-cluster #7("DO parameters"=w2788) -> (w2782:T17)
                                }
                                n397 = call "waveformparamsv2.vi"("command"="set", "Params in"=w2782) -> ()  [unwired: 3 in, 3 out]
                                }
                                frame 3, Default {
                                # "Remove True; Add True"
                                }
                                frame 0 {
                                # "remove False ; add False"
                                n398 = call "2pparameters.vi"("command"="get") -> ("params out"=w2801:T12)  [unwired: 1 in]
                                n399 = Unbundle By Name(w2801) -> ("autoshutter"=w2800:bool, "wavdet"=w2798:bool)
                                n400 = case shown="True" w2800 {
                                tunnel: w2799 -> [_ w2805]
                                tunnel: w2798 -> [_ w2804]
                                tunnel: [_ w2803] -> w2797
                                frame False {
                                }
                                frame True {
                                n401 = case shown="False" w2804 {
                                tunnel: w2805 -> [w2807 _]
                                tunnel: [w2806 _] -> w2803
                                frame False {
                                n402 = stacked-sequence {
                                tunnel: w2807 -> [w2809 w2816]
                                tunnel: [w2808 _] -> w2806
                                frame #0 {
                                n403 = call "waveformparamsv2.vi"("command"="get") -> ("Params out"=w2811:T17)  [unwired: 4 in, 2 out]
                                n404 = Unbundle By Name(w2811) -> ("DO parameters"=w2810:T20)
                                n405 = for {
                                tunnel: w2810 -> [w2815]
                                tunnel: w2809 -> [w2814] mode=indexing
                                tunnel: [w2813] -> w2808 mode=indexing
                                n406 = Index Array(array=w2815, index=w2814) -> (element=w2813:T21)
                                }
                                }
                                frame #1 {
                                n407 = for {
                                tunnel: w2816 -> [w2827] mode=indexing
                                w2826 = 0.0 ("padding value")
                                n408 = call "2pparameters.vi"("command"="get") -> ("params out"=w2824:T12)  [unwired: 1 in]
                                n409 = Unbundle By Name(w2824) -> ("srate"=w2821:sgl, "sAOxy"=w2823:i32)
                                n410 = To Double Precision Float(number=w2821) -> (double precision float=w2819:dbl)
                                n411 = To Double Precision Float(number=w2821) -> (double precision float=w2820:dbl)
                                n412 = To Double Precision Float(number=w2823) -> (double precision float=w2822:dbl)
                                n413 = Divide(x=w2820, y=w2822) -> (x/y=w2818:dbl)
                                n414 = call "replace DO wf param.vi"("Digital Freq (Hz)"=w2818, "Digital DC (%)"=100.0, "Digital phase"=w2826, "Sampling frequency (Hz)"=w2819, "Digital time offset (s)"=w2826, "index of DO wave"=w2827, "padding value"=w2826, "matlab wave file"=path "2Pshutter" ("matlab wave number")) -> ()  [unwired: 3 in]
                                }
                                }
                                }
                                }
                                frame True {
                                }
                                }
                                }
                                }
                                }
                                }
                              }
                              frame #7 {
                                # "... and add the actual 2p shutter waveform"
                                n415 = Build Array(w2832, w2831) -> (w2834:bool[])
                                n416 = Boolean Array To Number(Boolean array=w2834) -> (number=w2833:u32)
                                n417 = case shown="2" w2833 {
                                tunnel: w2830 -> [w2836 w2881 _ w2892]
                                tunnel: [_ w2882 _ w2890] -> w2829
                                frame 1 {
                                n418 = call "2pparameters.vi"("command"="get") -> ("params out"=w2843:T12)  [unwired: 1 in]
                                n419 = Unbundle By Name(w2843) -> ("wavdet"=w2844:bool, "sAOxy"=w2846:i32, "refwfsize"=w2847:dbl, "srate Img"=w2845:sgl)
                                n420 = call "waveformsDObuffer.vi"("command"="get") -> ("DO wf out"=w2839:digitalwaveform[])  [unwired: 1 in]
                                n421 = case shown="False" w2844 {
                                tunnel: [w2855 w2865] -> w2841
                                tunnel: w2845 -> [w2860 w2876]
                                tunnel: w2846 -> [w2854 w2869]
                                tunnel: w2847 -> [_ w2873]
                                frame False {
                                w2858 = u16 0 items=["unsigned binary", "offset binary", "2's complement"] ("data format (offset binary)")
                                n422 = Initialize Array(sgl 1.0, w2854) -> (w2851:sgl[])
                                n423 = Reciprocal(x=w2860) -> (1/x=w2861:sgl)
                                n424 = Bundle By Name("Y"=w2851, "dt"=w2861) -> (w2856:waveform(sgl))  [unwired: 1 in]
                                n425 = call-poly <vilib>:"Analog to Digital.vi"("data format (offset binary)"=w2858, "compress digital (T)"=TRUE, "full-scale range (pk-pk)"=1.0, "resolution (16 bit)"=1, "analog waveform"=w2856) -> ("digital waveform"=w2855:digitalwaveform)  [unwired: 3 in, 3 out]
                                }
                                frame True {
                                w2868 = u16 0 items=["unsigned binary", "offset binary", "2's complement"] ("data format (offset binary)")
                                n426 = To Double Precision Float(number=w2869) -> (double precision float=w2874:dbl)
                                n427 = Initialize Array(sgl 1.0, w2869) -> (w2862:sgl[])
                                n428 = Divide(x=w2873, y=w2874) -> (x/y=w2871:dbl)
                                n429 = Round Toward +Infinity(x=w2871) -> (ceil(x): smallest int >= x=w2872:dbl)
                                n430 = for {
                                N: w2872 -> [_]
                                tunnel: w2862 -> [w2878]
                                tunnel: [w2878] -> w2875 mode=concatenating
                                }
                                n431 = Reciprocal(x=w2876) -> (1/x=w2877:sgl)
                                n432 = Bundle By Name("Y"=w2875, "dt"=w2877) -> (w2866:waveform(sgl))  [unwired: 1 in]
                                n433 = call-poly <vilib>:"Analog to Digital.vi"("data format (offset binary)"=w2868, "compress digital (T)"=TRUE, "full-scale range (pk-pk)"=1.0, "resolution (16 bit)"=1, "analog waveform"=w2866) -> ("digital waveform"=w2865:digitalwaveform)  [unwired: 3 in, 3 out]
                                }
                                }
                                n434 = Array Size(array=w2836) -> (size(s)=w2835:i32)
                                n435 = for {
                                N: w2835 -> [_]
                                tunnel: w2841 -> [w2850]
                                shift-right: [w2848] -> w2837
                                shift-left: w2839 -> [w2849]
                                n436 = Build Array (concatenate)(w2849, w2850) -> (w2848:digitalwaveform[])
                                }
                                n437 = call "waveformsDObuffer.vi"("DO wf in"=w2837, "command"="set") -> ()  [unwired: 1 out]
                                }
                                frame 2 {
                                n438 = Sort 1D Array(array=w2881) -> (sorted array=w2880:i32[])
                                n439 = Reverse 1D Array(array=w2880) -> (reversed array=w2879:i32[])
                                n440 = for {
                                tunnel: w2879 -> [w2885] mode=indexing
                                tunnel: [w2884] -> w2882
                                n441 = call "waveformsDObuffer.vi"("command"="get") -> ("DO wf out"=w2887:digitalwaveform[])  [unwired: 1 in]
                                n442 = Delete From Array(array=w2887, length=1, index=w2885) -> (deleted portion=w2884:digitalwaveform[], array with subset deleted=w2883:digitalwaveform[])
                                n443 = call "waveformsDObuffer.vi"("DO wf in"=w2883, "command"="set") -> ()  [unwired: 1 out]
                                }
                                }
                                frame 3, Default {
                                }
                                frame 0 {
                                n444 = call "2pparameters.vi"("command"="get") -> ("params out"=w2894:T12)  [unwired: 1 in]
                                n445 = Unbundle By Name(w2894) -> ("autoshutter"=w2893:bool, "wavdet"=w2891:bool)
                                n446 = case shown="True" w2893 {
                                tunnel: w2892 -> [_ w2898]
                                tunnel: w2891 -> [_ w2897]
                                tunnel: [_ w2896] -> w2890
                                frame False {
                                }
                                frame True {
                                n447 = case shown="False" w2897 {
                                tunnel: w2898 -> [w2901 _]
                                tunnel: [w2900 _] -> w2896
                                frame False {
                                w2908 = u16 0 items=["unsigned binary", "offset binary", "2's complement"] ("data format (offset binary)")
                                n448 = call "2pparameters.vi"("command"="get") -> ("params out"=w2915:T12)  [unwired: 1 in]
                                n449 = call "waveformsDObuffer.vi"("command"="get") -> ("DO wf out"=w2902:digitalwaveform[])  [unwired: 1 in]
                                n450 = Unbundle By Name(w2915) -> ("sAOxy"=w2917:i32, "srate Img"=w2916:sgl)
                                n451 = Initialize Array(sgl 1.0, w2917) -> (w2903:sgl[])
                                n452 = Reciprocal(x=w2916) -> (1/x=w2910:sgl)
                                n453 = Bundle By Name("Y"=w2903, "dt"=w2910) -> (w2906:waveform(sgl))  [unwired: 1 in]
                                n454 = call-poly <vilib>:"Analog to Digital.vi"("data format (offset binary)"=w2908, "compress digital (T)"=TRUE, "full-scale range (pk-pk)"=1.0, "resolution (16 bit)"=1, "analog waveform"=w2906) -> ("digital waveform"=w2913:digitalwaveform)  [unwired: 3 in, 3 out]
                                n455 = for {
                                tunnel: w2913 -> [w2922]
                                tunnel: w2901 -> [w2919] mode=indexing
                                tunnel: [w2918] -> w2900 mode=indexing
                                shift-right: [w2920] -> w2899
                                shift-left: w2902 -> [w2921]
                                n456 = Index Array(array=w2921, index=w2919) -> (element=w2918:digitalwaveform)
                                n457 = Replace Array Subset(array=w2921, new element=w2922, index=w2919) -> (w2920:digitalwaveform[])
                                }
                                n458 = call "waveformsDObuffer.vi"("DO wf in"=w2899, "command"="set") -> ()  [unwired: 1 out]
                                }
                                frame True {
                                }
                                }
                                }
                                }
                                }
                                }
                              }
                              frame #8 {
                                # "Calculate lifetime timestamp waveform"
                                n459 = Build Array(w2926, w2925) -> (w2928:bool[])
                                n460 = Boolean Array To Number(Boolean array=w2928) -> (number=w2927:u32)
                                n461 = case shown="0" w2927 {
                                tunnel: w2924 -> [_ w2954 _ w2966]
                                tunnel: [_ w2953 _ w2964] -> w2923
                                frame 1 {
                                w2941 = 0.0 ("DOtab")
                                n462 = call "2pparameters.vi"("command"="get") -> ("params out"=w2939:T12)  [unwired: 1 in]
                                n463 = call "waveformparamsv2.vi"("command"="get") -> ("Params out"=w2949:T17)  [unwired: 4 in, 2 out]
                                n464 = Unbundle By Name(w2949) -> ("DO parameters"=w2947:T20)
                                n465 = Unbundle By Name(w2939) -> ("srate"=w2936:sgl, "sAOxy"=w2938:i32)
                                n466 = To Double Precision Float(number=w2936) -> (double precision float=w2934:dbl)
                                n467 = To Double Precision Float(number=w2936) -> (double precision float=w2935:dbl)
                                n468 = To Double Precision Float(number=w2938) -> (double precision float=w2930:dbl)
                                n469 = Divide(x=w2935, y=w2930) -> (x/y=w2937:dbl)
                                n470 = Index Array(array=w2947, index=0) -> (element=w2946:T21)
                                n471 = Divide(x=1.0 ("Digital DC (%)"), y=w2930) -> (x/y=w2932:dbl)
                                n472 = Multiply(x=100.0, y=w2932) -> (x*y=w2929:dbl)
                                n473 = Bundle By Name(cluster=w2946, "Digital DC (%)"=w2929, "Digital phase"=w2941, "Digital Freq (Hz)"=w2937, "Sampling frequency (Hz)"=w2934, "Digital time offset (s)"=w2941, "padding value"=0.0, "matlab wave file"=path "LT", "DOtab"=0.0) -> (w2944:T21)
                                n474 = Build Array(w2944) -> (w2943:T20)
                                n475 = call "waveformparamsv2.vi"("command"="add DO", "add DO"=w2943) -> ()  [unwired: 3 in, 3 out]
                                }
                                frame 2 {
                                n476 = call "waveformparamsv2.vi"("command"="get") -> ("Params out"=w2956:T17)  [unwired: 4 in, 2 out]
                                n477 = in-place {
                                in-place-border: w2954 -> [w2960]
                                in-place-border: [w2959] -> w2953
                                n478 = in-place-cluster #8(w2956) -> ("DO parameters"=w2962:T20)
                                n479 = Delete From Array(array=w2962, length=1, index=w2960) -> (deleted portion=w2959:T20, array with subset deleted=w2961:T20)
                                n480 = in-place-cluster #8("DO parameters"=w2961) -> (w2955:T17)
                                }
                                n481 = call "waveformparamsv2.vi"("command"="set", "Params in"=w2955) -> ()  [unwired: 3 in, 3 out]
                                }
                                frame 3, Default {
                                }
                                frame 0 {
                                n482 = local read "Measurement"() -> (w2968:T4)
                                n483 = To Unsigned Long Integer(number=w2968) -> (unsigned 32bit integer=w2967:u32)
                                n484 = case shown="5..7" w2967 {
                                tunnel: w2966 -> [_ w2970]
                                tunnel: [_ w2969] -> w2965
                                frame 0..4, Default {
                                }
                                frame 5..7 {
                                n485 = stacked-sequence {
                                tunnel: w2970 -> [w2972 w2981]
                                tunnel: [w2971 _] -> w2969
                                frame #0 {
                                n486 = call "waveformparamsv2.vi"("command"="get") -> ("Params out"=w2974:T17)  [unwired: 4 in, 2 out]
                                n487 = Unbundle By Name(w2974) -> ("DO parameters"=w2975:T20)
